vi "Asyncronous launcher.vi"(0 "Master serial cluster":T2, 5 "ROB Serial cluster":T1, 7 "GPS Serial cluster":T1, 9 "Sniffer serial cluster":T1, 11 "error in":errorcluster) -> (4 "MasterSerial Refnum":refnum<vi>, 6 "SnifferSerial Refnum":refnum<vi>, 8 "GPSSerial Refnum":refnum<vi>, 10 "ROBSerial Refnum":refnum<vi>, 15 "error out":errorcluster)   [LabVIEW 2016]
panel:
  # "This VI launches the serial port monitors and loggers asynchronously.\nIt is of great importance that the CRT Controller is stopped in a safe manner,\nas these VIs can ONLY be stopped by sending a TRUE on the stop-notifier."
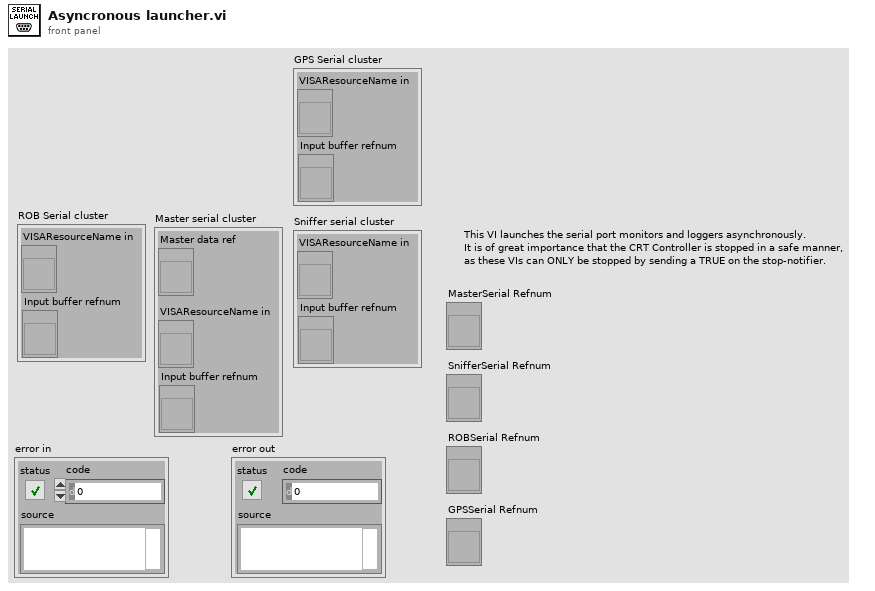
[diagram p1: front panel]
types:
  T1 = cluster{"VISAResourceName in":refnum<vi>, "Input buffer refnum":refnum<vi>}
  T2 = cluster{"Master data ref":refnum<vi>, "VISAResourceName in":refnum<vi>, "Input buffer refnum":refnum<vi>}
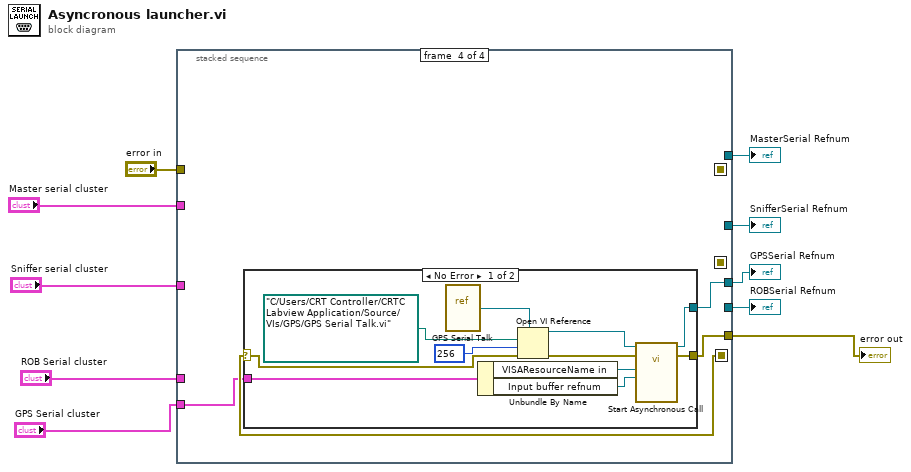
[diagram p0: block diagram]
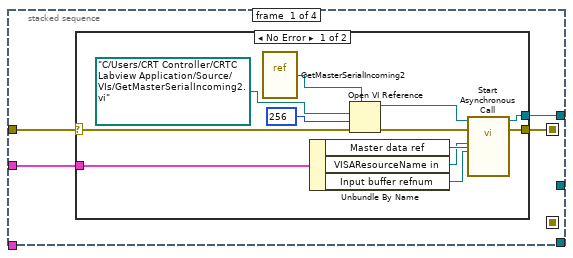
[diagram p2: hidden frame]
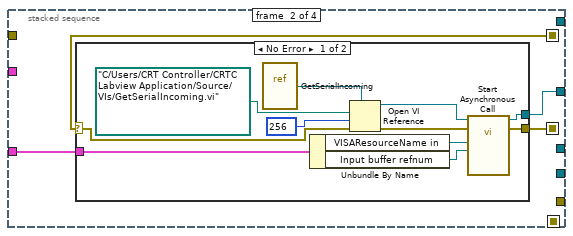
[diagram p4: hidden frame]
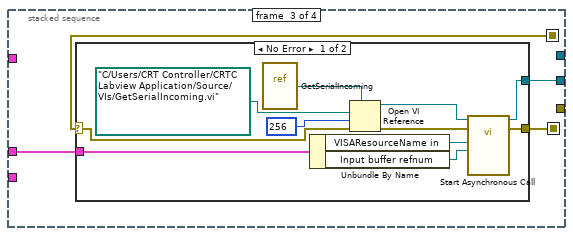
[diagram p6: hidden frame]
diagram:
  n1 = stacked-sequence {
    seq-local: [w13 _ _ _] -> [_ w31 _ _]
    seq-local: [_ w29 _ _] -> [_ _ w47 _]
    seq-local: [_ _ w44 _] -> [_ _ _ w63]
    tunnel: "Master serial cluster" -> [w14 _ _ _]
    tunnel: "error in" -> [w12 _ _ _]
    tunnel: "Sniffer serial cluster" -> [_ w30 _ _]
    tunnel: "ROB Serial cluster" -> [_ _ w46 _]
    tunnel: [_ _ w45 _] -> w7
    tunnel: [w11 _ _ _] -> w6
    tunnel: [_ w28 _ _] -> w5
    tunnel: [_ _ _ w62] -> w4
    tunnel: [_ _ _ w61] -> w1
    tunnel: "GPS Serial cluster" -> [_ _ _ w60]
    frame #0 {
      n2 = case shown="No Error" w12 {
        selector: w12 -> [w17 w27]
        tunnel: w14 -> [w21 _]
        tunnel: [w16 w27] -> w13
        tunnel: [w15 _] -> w11
        frame No Error {
          n3 = vi-ref "GetMasterSerialIncoming2.vi"() -> (w24:refnum<vi>)
          n4 = Unbundle By Name(w21) -> ("Master data ref"=w20:refnum<vi>, "VISAResourceName in"=w19:refnum<vi>, "Input buffer refnum"=w18:refnum<vi>)
          n5 = Open VI Reference(type specifier VI Refnum (for type only)=w24, vi path=path "C:/Users/CRT Controller/CRTC Labview Application/Source/VIs/GetMasterSerialIncoming2.vi", options=256, error in (no error)=w17) -> (vi reference=w23:refnum<vi>, error out=w22:errorcluster)  [unwired: 2 in]
          n6 = call-by-ref "Start Asynchronous Call"(reference=w23, error in=w22, "Master data ref"=w20, "Input buffer refnum"=w18, "VISAResourceName in"=w19) -> (reference out=w15:refnum<vi>, error out=w16:errorcluster)  [unwired: 8 in, 1 out]
        }
        frame Error {
        }
      }
    }
    frame #1 {
      n7 = case shown="No Error" w31 {
        selector: w31 -> [w34 w43]
        tunnel: w30 -> [w37 _]
        tunnel: [w33 w43] -> w29
        tunnel: [w32 _] -> w28
        frame No Error {
          n8 = vi-ref "GetSerialIncoming.vi"() -> (w40:refnum<vi>)
          n9 = Unbundle By Name(w37) -> ("VISAResourceName in"=w36:refnum<vi>, "Input buffer refnum"=w35:refnum<vi>)
          n10 = Open VI Reference(type specifier VI Refnum (for type only)=w40, vi path=path "C:/Users/CRT Controller/CRTC Labview Application/Source/VIs/GetSerialIncoming.vi", options=256, error in (no error)=w34) -> (vi reference=w39:refnum<vi>, error out=w38:errorcluster)  [unwired: 2 in]
          n11 = call-by-ref "Start Asynchronous Call"(reference=w39, error in=w38, "Input buffer refnum"=w35, "VISAResourceName in"=w36) -> (reference out=w32:refnum<vi>, error out=w33:errorcluster)  [unwired: 9 in, 1 out]
        }
        frame Error {
        }
      }
    }
    frame #2 {
      n12 = case shown="No Error" w47 {
        selector: w47 -> [w50 w59]
        tunnel: w46 -> [w53 _]
        tunnel: [w49 w59] -> w44
        tunnel: [w48 _] -> w45
        frame No Error {
          n13 = vi-ref "GetSerialIncoming.vi"() -> (w56:refnum<vi>)
          n14 = Unbundle By Name(w53) -> ("VISAResourceName in"=w52:refnum<vi>, "Input buffer refnum"=w51:refnum<vi>)
          n15 = Open VI Reference(type specifier VI Refnum (for type only)=w56, vi path=path "C:/Users/CRT Controller/CRTC Labview Application/Source/VIs/GetSerialIncoming.vi", options=256, error in (no error)=w50) -> (vi reference=w55:refnum<vi>, error out=w54:errorcluster)  [unwired: 2 in]
          n16 = call-by-ref "Start Asynchronous Call"(reference=w55, error in=w54, "Input buffer refnum"=w51, "VISAResourceName in"=w52) -> (reference out=w48:refnum<vi>, error out=w49:errorcluster)  [unwired: 9 in, 1 out]
        }
        frame Error {
        }
      }
    }
    frame #3 {
      n17 = case shown="No Error" w63 {
        selector: w63 -> [w68 w75]
        tunnel: w60 -> [w71 _]
        tunnel: [w67 w75] -> w62
        tunnel: [w66 _] -> w61
        frame No Error {
          n18 = vi-ref "GPS Serial Talk.vi"() -> (w64:refnum<vi>)
          n19 = Unbundle By Name(w71) -> ("VISAResourceName in"=w70:refnum<vi>, "Input buffer refnum"=w69:refnum<vi>)
          n20 = Open VI Reference(type specifier VI Refnum (for type only)=w64, vi path=path "C:/Users/CRT Controller/CRTC Labview Application/Source/VIs/GPS/GPS Serial Talk.vi", options=256, error in (no error)=w68) -> (vi reference=w65:refnum<vi>, error out=w72:errorcluster)  [unwired: 2 in]
          n21 = call-by-ref "Start Asynchronous Call"(reference=w65, error in=w72, "Input buffer refnum"=w69, "VISAResourceName in"=w70) -> (reference out=w66:refnum<vi>, error out=w67:errorcluster)  [unwired: 9 in, 1 out]
        }
        frame Error {
        }
      }
    }
  }
  "error out" <- w4
  "ROBSerial Refnum" <- w7
  "MasterSerial Refnum" <- w6
  "SnifferSerial Refnum" <- w5
  "GPSSerial Refnum" <- w1
